vi "PRO8.vi"() -> ()   [LabVIEW 2019]
uses:
  <vilib>/Instr/_visa.llb/VISA Open Access Mode.ctl
  <vilib>/Instr/_visa.llb/VISA Configure Serial Port (Instr).vi
panel:
  out "return count 2":u32
  out "read buffer 2":string
  out "return count":u32
  out "read buffer":string
  out "error out":errorcluster
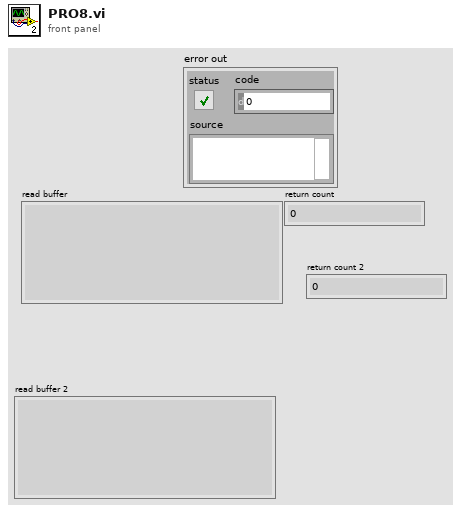
[diagram p1: front panel]
types:
  T1 = typedef "VISA Open Access Mode.ctl" = u32
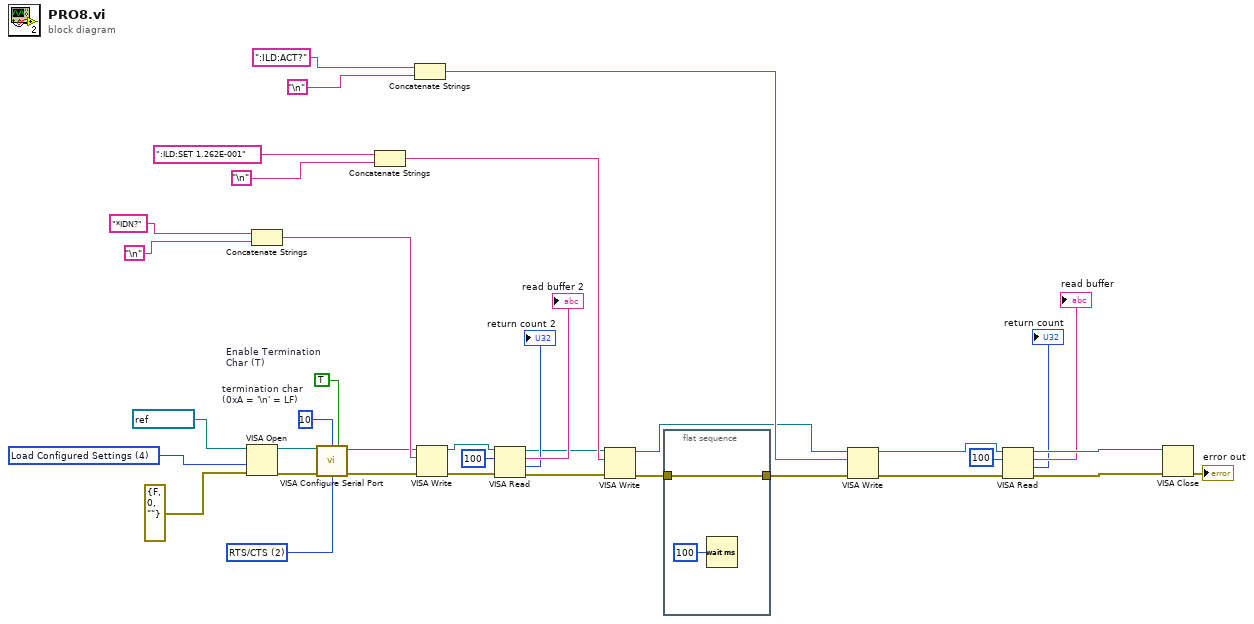
[diagram p0: block diagram]
diagram:
  w20 = u16 2 items=["None", "XON/XOFF", "RTS/CTS", "XON/XOFF & RTS/CTS", "DTR/DSR", "XON/XOFF & DTR/DSR"] ("flow control (0:none)")
  w21 = u8 10  # termination char (0xA = '\n' = LF)
  w22 = TRUE  # Enable Termination Char (T)
  w34 = T1 4 items=["VISA Defaults"=0, "Exclusive Lock"=1, "Load Configured Settings"=4] ("Access Mode")
  n1 = VISA Open(access mode=w34, error in (no error)=errorcluster {"status"=FALSE, "code"=0, "source"=""}, VISA resource name=refnum<visa-resource-name> "COM4") -> (VISA resource name=w23:refnum<visa-resource-name>, error out=w26:errorcluster)  [unwired: 2 in]
  n2 = Concatenate Strings("*IDN?" ("write buffer"), "\n") -> (w32:string)
  n3 = call-poly "VISA Configure Serial Port"("VISA resource name"=w23, "termination char\n(0xA = '\\n' = LF)"=w21, "Enable Termination\nChar (T)"=w22, "error in (no error)"=w26, "flow control (0:none)"=w20) -> ("VISA resource name out"=w24:refnum<visa-resource-name>, "error out"=w25:errorcluster)  [unwired: 9 in]
  n4 = Concatenate Strings(":ILD:SET 1.262E-001" ("write buffer"), "\n") -> (w17:string)
  n5 = Concatenate Strings(":ILD:ACT?" ("write buffer"), "\n") -> (w4:string)
  n6 = VISA Write(VISA resource name=w24, write buffer=w32, error in (no error)=w25) -> (VISA resource name out=w12:refnum<visa-resource-name>, error out=w13:errorcluster)  [unwired: 1 out]
  n7 = VISA Read(VISA resource name=w12, byte count=u32 100, error in (no error)=w13) -> (VISA resource name out=w11:refnum<visa-resource-name>, read buffer=→"read buffer 2":string, return count=→"return count 2":u32, error out=w10:errorcluster)
  n8 = VISA Write(VISA resource name=w11, write buffer=w17, error in (no error)=w10) -> (VISA resource name out=w3:refnum<visa-resource-name>, error out=w9:errorcluster)  [unwired: 1 out]
  n9 = flat-sequence {
    tunnel: [w38] -> w6
    tunnel: w9 -> [w38]
    frame #0 {
      n10 = Wait (ms)(milliseconds to wait=u32 100) -> ()  [unwired: 1 out]
    }
  }
  n11 = VISA Write(VISA resource name=w3, write buffer=w4, error in (no error)=w6) -> (VISA resource name out=w2:refnum<visa-resource-name>, error out=w5:errorcluster)  [unwired: 1 out]
  n12 = VISA Read(VISA resource name=w2, byte count=u32 100, error in (no error)=w5) -> (VISA resource name out=w31:refnum<visa-resource-name>, read buffer=→"read buffer":string, return count=→"return count":u32, error out=w30:errorcluster)
  n13 = VISA Close(VISA resource name=w31, error in (no error)=w30) -> (error out=→"error out":errorcluster)
